vi "Get DMM Measurement.vi"(3 "error in":errorcluster, 4 "DMM Model":T1, 5 "DMM Address":refnum<visa-resource-name>="GPIB0::5::INSTR") -> (0 "error out":errorcluster, 1 "Measurement":dbl, 2 "VISA resource name out":refnum<visa-resource-name>)   [LabVIEW 2020]
uses:
  Typedefs/DMM Models Control.ctl
  <instrlib>/Agilent 34405/Agilent 34405.lvlib
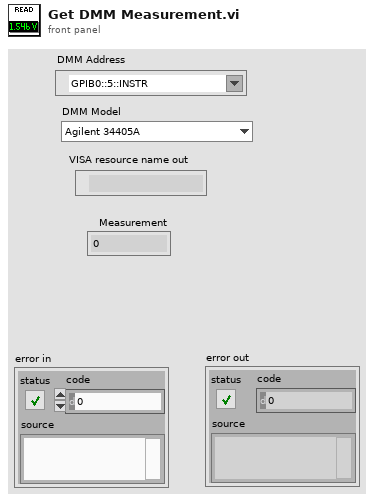
[diagram p1: front panel]
types:
  T1 = typedef "DMM Models Control.ctl" = enum16{"Agilent 34405A"}
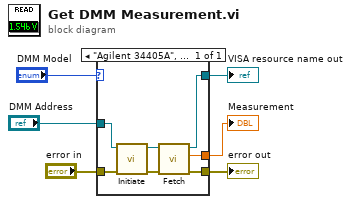
[diagram p0: block diagram]
diagram:
  n1 = case shown="\"Agilent 34405A\", Default" "DMM Model" {
    tunnel: "DMM Address" -> [w11]
    tunnel: "error in" -> [w10]
    tunnel: [w9] -> w3
    tunnel: [w8] -> w2
    tunnel: [w7] -> w1
    frame "Agilent 34405A", Default {
      n2 = call <instrlib>:"Initiate.vi"("error in (no error)"=w10, "VISA resource name"=w11) -> ("error out"=w13:errorcluster, "VISA resource name out"=w12:refnum<visa-resource-name>)  [unwired: 8 out]
      n3 = call <instrlib>:"Fetch.vi"("error in (no error)"=w13, "VISA resource name"=w12) -> ("error out"=w8:errorcluster, "Measurement"=w7:dbl, "VISA resource name out"=w9:refnum<visa-resource-name>)  [unwired: 7 out]
    }
  }
  "error out" <- w2
  "VISA resource name out" <- w3
  "Measurement" <- w1
